vi "Get Number Text.vi"(6 "LV Type":variant, 8 "error in (no error)":errorcluster, 10 "Offset":i32, 11 "JSON":string) -> (0 "error out":errorcluster, 1 "Offset past match":i32, 2 "Number Text":string, 4 "JSON Value Type":T1)   [LabVIEW 2020, in "JSONtext.lvlib"]
uses:
  <vilib>/JDP Science/JSONtext/JSONtext.lvlib
  <vilib>/JDP Science/JSONtext/JSON Value Type.ctl
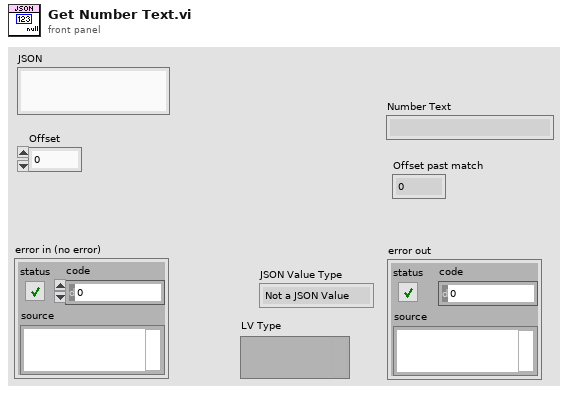
[diagram p1: front panel]
types:
  T1 = typedef "JSONtext.lvlib/JSON Value Type.ctl" = enum16{"Not a JSON Value", "JSON Object", "JSON Array", "String", "Number", "true", "false", "null"}
  T2 = typedef "JSONtext.lvlib/Parsing State.ctl" = enum16{"Parser Error", "Object", "Array", "String", "Number/Other", "Leading Whitespace", "Object end", "Array end", "Value end"}
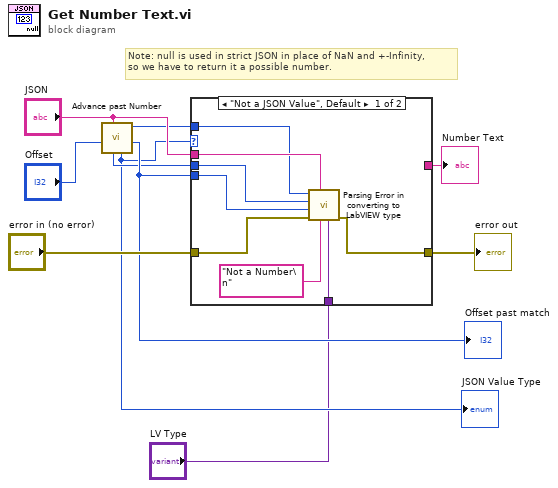
[diagram p0: block diagram]
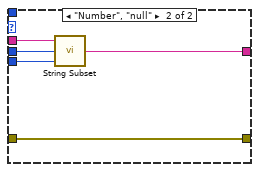
[diagram p2: hidden frame]
diagram:
  # "Note: null is used in strict JSON in place of NaN and +-Infinity,\nso we have to return it a possible number."
  n1 = call <vilib>:"Advance past Number.vi"("JSON"="JSON", "Offset (0)"="Offset") -> ("Offset past match"=w5:i32, "Parser State"=w2:T2, "JSON Value Type"=w3:T1, "Value start out"=w4:i32)  [unwired: 5 in, 1 out]
  "Offset past match" <- w5
  "JSON Value Type" <- w3
  n2 = case shown="\"Not a JSON Value\", Default" w3 {
    tunnel: "JSON" -> [w16 w23]
    tunnel: [w18 w19] -> w8
    tunnel: "error in (no error)" -> [w17 w19]
    tunnel: [_ w20] -> w6
    tunnel: w4 -> [w15 w22]
    tunnel: w5 -> [w14 w21]
    tunnel: w2 -> [w13 _]
    tunnel: "LV Type" -> [w11 _]
    frame "Not a JSON Value", Default {
      n3 = call <vilib>:"Parsing Error in converting to LabVIEW type.vi"("LV Type"=w11, "initial string"="Not a Number\n", "JSON"=w16, "error in (no error)"=w17, "Offset past match"=w14, "Value start"=w15, "State"=w13) -> ("error out"=w18:errorcluster)  [unwired: 4 in]
    }
    frame "Number", "null" {
      n4 = call <vilib>:"String Subset.vi"("Offset past End"=w21, "Start offset"=w22, "JSON"=w23) -> ("substring"=w20:string)  [unwired: 2 in]
    }
  }
  "error out" <- w8
  "Number Text" <- w6
